vi "Initialise.vi"(8 "error in (no error)":errorcluster, 10 "Instrument Ref":string, 11 "NI 6514 in":refnum<class "NI 6514.lvclass">) -> (0 "error out":errorcluster, 3 "NI 6514 out":refnum<class "NI 6514.lvclass">)   [LabVIEW 2021, in "Concrete.lvlib" / "NI 6514.lvclass"]
uses:
  NI 6514.lvclass
  NI 6514.lvclass/NI 6514.ctl
  <vilib>/DAQmx/create/channels.llb/DAQmx Create Channel (DO-Digital Output).vi
  Harware Abstraction/DIO/DIO.lvclass
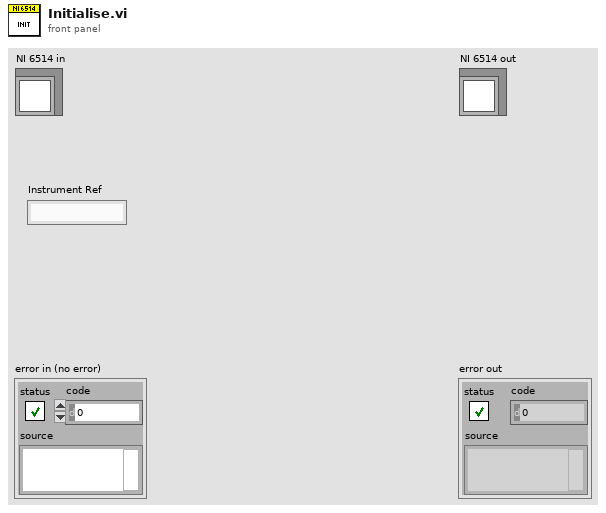
[diagram p1: front panel]
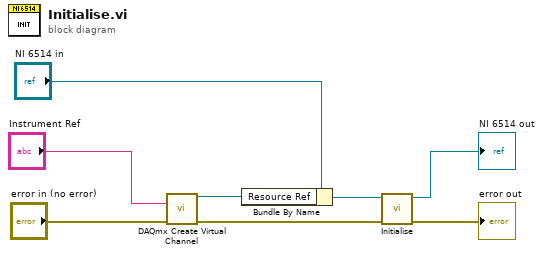
[diagram p0: block diagram]
diagram:
  n1 = call-poly <vilib>:"DAQmx Create Virtual Channel.vi"("lines"="Instrument Ref", "error in"="error in (no error)") -> ("task out"=w2:refnum<k21>, "error out"=w5:errorcluster)  [unwired: 12 in]
  n2 = Bundle By Name(cluster="NI 6514 in", "Resource Ref"=w2) -> (w1:refnum<class "NI 6514.lvclass">)
  n3 = call-parent "Initialise.vi"("error in (no error)"=w5, "Instrument in"=w1) -> ("error out"=→"error out":errorcluster, "Instrument out"=→"NI 6514 out":refnum<class "NI 6514.lvclass">)  [unwired: 8 in]
